vi "Check Value.vi"(6 "Coerce Value? (F)":bool, 7 "Column Configuration":refnum<class "Column Configuration.lvclass">, 8 "error in (no error)":errorcluster, 9 "Value Type":refnum<class "Value Type.lvclass">, 10 "Value":variant, 11 "Unique in":refnum<class "Unique.lvclass">) -> (0 "error out":errorcluster, 2 "Value Out":variant, 3 "Unique out":refnum<class "Unique.lvclass">)   [LabVIEW 2020, in "Composed Columns.lvlib" / "Unique.lvclass"]
uses:
  Unique.lvclass
  Value Type/Value Type.lvclass
  Database Libraries/Database Interfaces/Database Interface Class/Database Interface.lvclass
  Column Interface/Column Configuration Interface Class/Column Configuration.lvclass
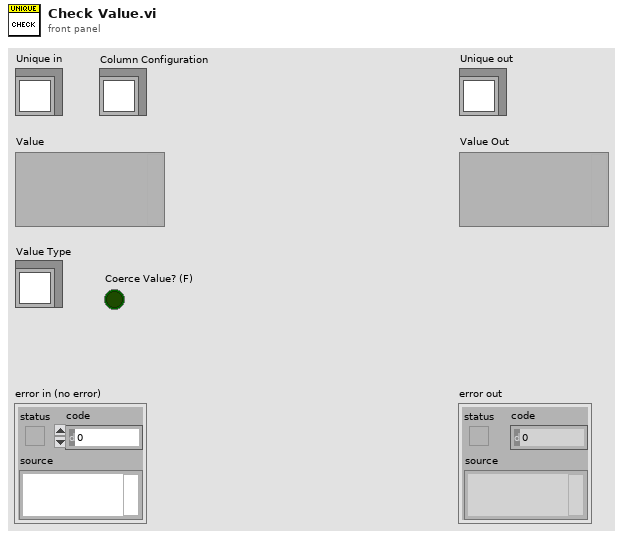
[diagram p1: front panel]
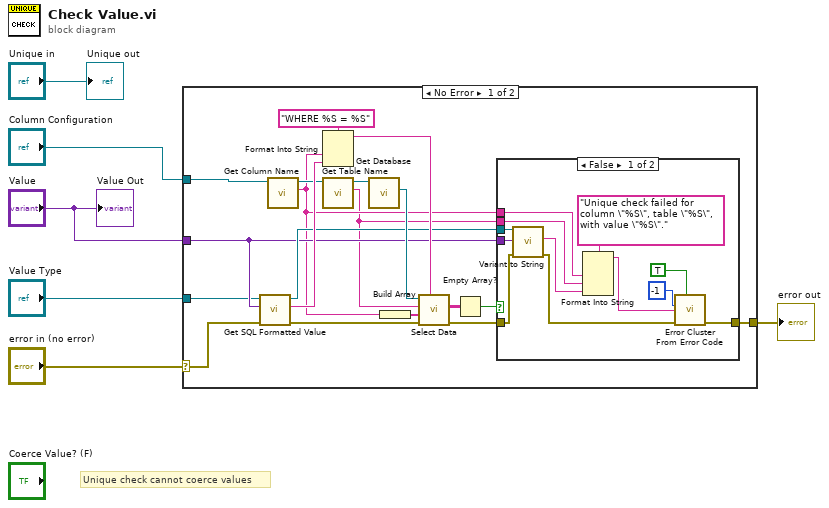
[diagram p0: block diagram]
diagram:
  # "Unique check cannot coerce values"
  n1 = case shown="No Error" "error in (no error)" {
    selector: "error in (no error)" -> [w8 w39]
    tunnel: [w13 w39] -> w5
    tunnel: "Value Type" -> [w7 _]
    tunnel: "Value" -> [w11 _]
    tunnel: "Column Configuration" -> [w20 _]
    frame No Error {
      n2 = call-dynamic "Get SQL Formatted Value.vi"("error in (no error)"=w8, "Value"=w11, "Value Type in"=w7) -> ("error out"=w17:errorcluster, "SQL Formatted Value"=w24:string, "Value Type out"=w12:refnum<class "Value Type.lvclass">)  [unwired: 6 in]
      n3 = call-dynamic "Get Column Name.vi"("Column Configuration in"=w20) -> ("Column Name"=w10:string, "Column Configuration out"=w19:refnum<class "Column Configuration.lvclass">)  [unwired: 8 in, 1 out]
      n4 = Format Into String(format string="WHERE %S = %S", w10, w24) -> (resulting string=w23:string)  [unwired: 2 in, 1 out]
      n5 = call-dynamic "Get Table Name.vi"("Column Configuration in"=w19) -> ("Table Name"=w9:string, "Column Configuration out"=w18:refnum<class "Column Configuration.lvclass">)  [unwired: 8 in, 1 out]
      n6 = call-dynamic "Get Database.vi"("Column Configuration in"=w18) -> ("Database"=w21:refnum<class "Database Interface.lvclass">)  [unwired: 8 in, 2 out]
      n7 = Build Array(w10) -> (w22:string[])
      n8 = call-dynamic "Select Data.vi"("WHERE Statement"=w23, "error in (no error)"=w17, "Columns"=w22, "Table"=w9, "Database Interface in"=w21) -> ("error out"=w14:errorcluster, "Data"=w16:string[][])  [unwired: 4 in, 1 out]
      n9 = Empty Array?(array=w16) -> (empty?=w15:bool)
      n10 = case shown="False" w15 {
        tunnel: w14 -> [w30 w38]
        tunnel: [w33 w38] -> w13
        tunnel: w12 -> [w32 _]
        tunnel: w11 -> [w31 _]
        tunnel: w10 -> [w27 _]
        tunnel: w9 -> [w26 _]
        frame False {
          n11 = call-dynamic "Variant to String.vi"("error in (no error)"=w30, "Variant"=w31, "Value Type in"=w32) -> ("error out"=w29:errorcluster, "String"=w28:string)  [unwired: 6 in, 1 out]
          n12 = Format Into String(format string="Unique check failed for column \"%S\", table \"%S\", with value \"%S\".", w27, w26, w28) -> (resulting string=w37:string)  [unwired: 2 in, 1 out]
          n13 = call <vilib>:"Error Cluster From Error Code.vi"("show call chain? (False)"=TRUE, "error in (no error)"=w29, "error message (\"\")"=w37, "error code (0)"=-1) -> ("error out"=w33:errorcluster)  [unwired: 5 in]
        }
        frame True {
        }
      }
    }
    frame Error {
    }
  }
  "error out" <- w5
  "Unique out" <- "Unique in"
  "Value Out" <- "Value"
